vi "VsEP-Next Atten.vi"(0 "Runtime":T1, 11 "error in (no error)":errorcluster) -> (4 "Runtime out":T1, 14 "Finished":bool, 15 "error out":errorcluster)   [LabVIEW 2020]
uses:
  Typedefs/VsEP-Runtime Data.ctl
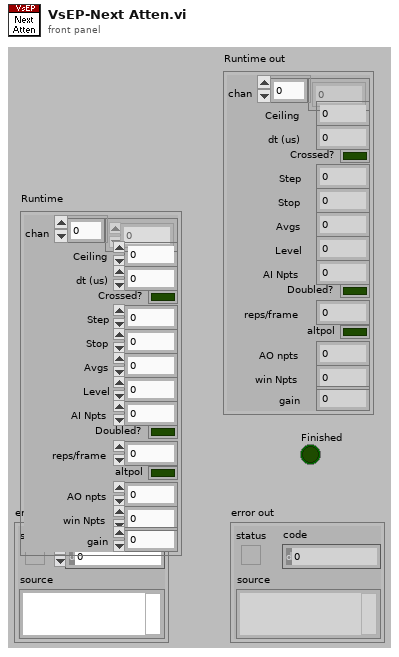
[diagram p1: front panel]
types:
  T1 = typedef "VsEP-Runtime Data.ctl" = cluster{"chan":i32[], "Ceiling":dbl, "dt (us)":dbl, "Crossed?":bool, "Step":dbl, "Stop":i32, "Avgs":i32, "Level":dbl, "AI Npts":i32, "Doubled?":bool, "reps/frame":i32, "altpol":bool, "AO npts":i32, "win Npts":i32, "gain":dbl}
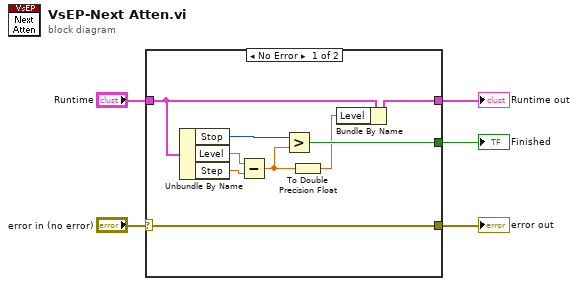
[diagram p0: block diagram]
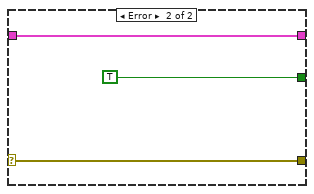
[diagram p2: hidden frame]
diagram:
  n1 = case shown="No Error" "error in (no error)" {
    selector: "error in (no error)" -> [w11 w16]
    tunnel: "Runtime" -> [w7 w17]
    tunnel: [w12 TRUE] -> w3
    tunnel: [w10 w17] -> w2
    tunnel: [w11 w16] -> w1
    frame No Error {
      n2 = Unbundle By Name(w7) -> ("Stop"=w14:i32, "Level"=w6:dbl, "Step"=w8:dbl)
      n3 = Subtract(x=w6, y=w8) -> (x-y=w13:dbl)
      n4 = Greater?(x=w14, y=w13) -> (0:w12:bool)
      n5 = To Double Precision Float(number=w13) -> (double precision float=w9:dbl)
      n6 = Bundle By Name(cluster=w7, "Level"=w9) -> (w10:T1)
    }
    frame Error {
    }
  }
  "error out" <- w1
  "Runtime out" <- w2
  "Finished" <- w3
